vi "Restore Front Panel Window Position From File.vi"(8 "error in (no error)":errorcluster, 11 "Actor in":refnum<class "Actor.lvclass">) -> (0 "error out":errorcluster)   [LabVIEW 2021, in "Actor.lvclass"]
uses:
  Actor.lvclass
  Actor.lvclass/Actor.ctl
  <vilib>/Utility/miscctls.llb/LVRectTypeDef.ctl
  <userlib>/_OpenG.lib/variantconfig/variantconfig.llb/openg_variant_configuration_file.lvlib
  <vilib>/Utility/config.llb/NI_LVConfig.lvlib
  <userlib>/_OpenG.lib/file/file.llb/openg_file.lvlib
  <userlib>/_OpenG.lib/file/file.llb/File Exists - Scalar__ogtk.vi
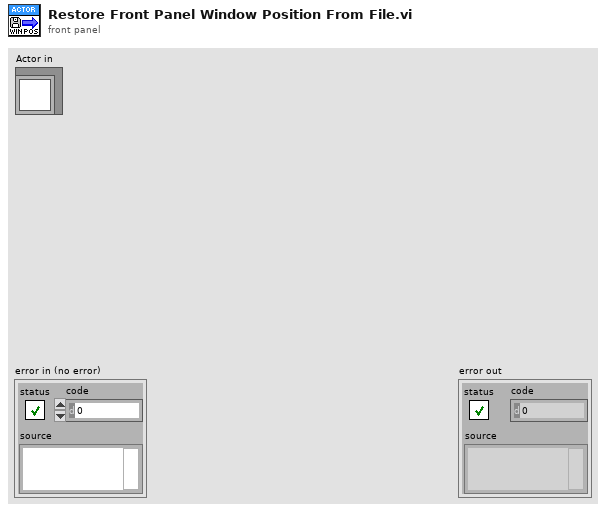
[diagram p1: front panel]
types:
  T1 = typedef "LVRectTypeDef.ctl" = cluster{"Left":i16, "Top":i16, "Right":i16, "Bottom":i16}
  T2 = typedef "NI_LVConfig.lvlib/Config Data RefNum.ctl" = refnum<k1>
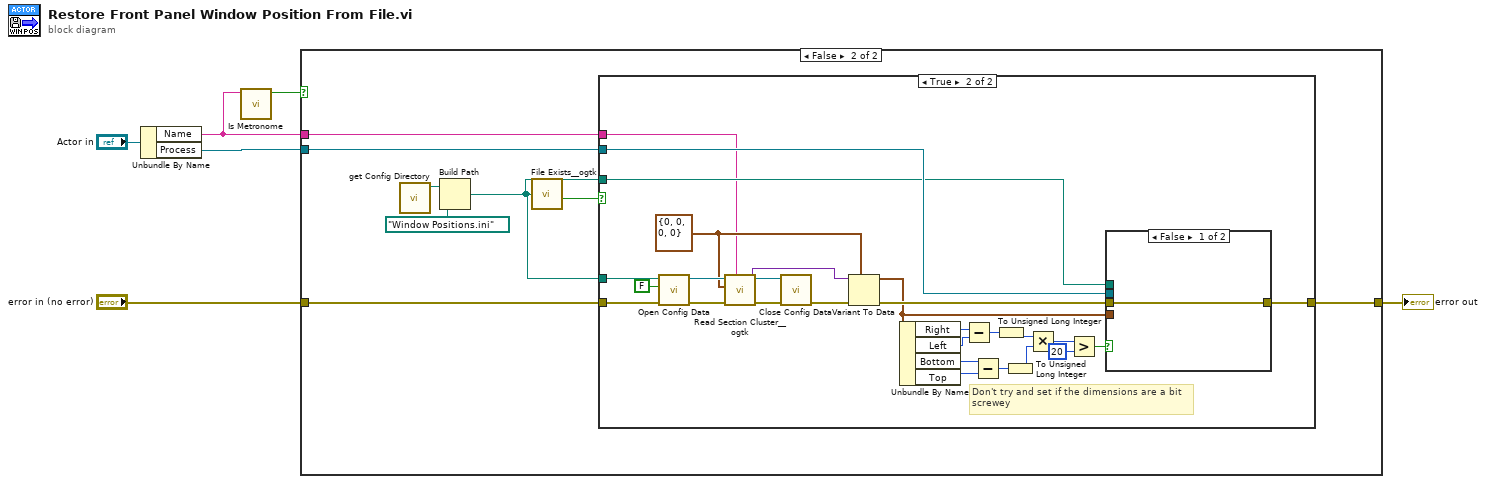
[diagram p0: block diagram]
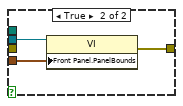
[diagram p4: hidden frame]
diagram:
  n1 = Unbundle By Name("Actor in") -> ("Name"=w1:string, "Process"=w5:refnum<vi>)
  n2 = call "Is Metronome.vi"("Actor Name"=w1) -> ("Is Metronome"=w2:bool)  [unwired: 10 in]
  n3 = case shown="False" w2 {
    tunnel: "error in (no error)" -> [w7 w9]
    tunnel: w5 -> [_ w15]
    tunnel: [w7 w13] -> w3
    tunnel: w1 -> [_ w8]
    frame True {
      # "Do not bother loading positions of Metronomes"
    }
    frame False {
      n4 = call "get Config Directory.vi"() -> ("Config Dir"=w10:path)  [unwired: 11 in]
      n5 = Build Path(base path=w10, name or relative path=path "Window Positions.ini" ("configuration file path")) -> (appended path=w11:path)
      n6 = call-poly <userlib>:"File Exists__ogtk.vi"("file path"=w11) -> ("exists"=w12:bool)  [unwired: 6 in, 1 out]
      n7 = case shown="True" w12 {
        tunnel: w9 -> [w16 w43]
        tunnel: w15 -> [_ w33]
        tunnel: [w16 w32] -> w13
        tunnel: w11 -> [_ w21]
        tunnel: w11 -> [_ w18]
        tunnel: w8 -> [_ w17]
        frame False {
        }
        frame True {
          w35 = T1 {"Left"=0, "Top"=0, "Right"=0, "Bottom"=0} ("Front Panel Window:Panel Bounds")
          # "Don't try and set if the dimensions are a bit screwey"
          n8 = call <vilib>:"Open Config Data.vi"("error in (no error)"=w43, "create file if necessary (T)"=FALSE, "configuration file path"=w21) -> ("error out"=w37:errorcluster, "refnum"=w38:T2)  [unwired: 6 in, 1 out]
          n9 = call <userlib>:"Read Section Cluster__ogtk.vi"("section (optional)"=w17, "error in (no error)"=w37, "Section Formatted Cluster Type"=w35, "refnum"=w38) -> ("error out"=w41:errorcluster, "Section Formatted Cluster"=w36:variant, "dup refnum"=w40:T2)  [unwired: 3 in, 2 out]
          n10 = call <vilib>:"Close Config Data.vi"("error in (no error)"=w41, "refnum"=w40) -> ("error out"=w42:errorcluster)  [unwired: 8 in, 1 out]
          n11 = Variant To Data(error in=w42, type=w35, Variant=w36) -> (data=w31:T1, error out=w34:errorcluster)
          n12 = Unbundle By Name(w31) -> ("Right"=w30:i16, "Left"=w29:i16, "Bottom"=w28:i16, "Top"=w27:i16)
          n13 = Subtract(x=w30, y=w29) -> (x-y=w26:i16)
          n14 = Subtract(x=w28, y=w27) -> (x-y=w25:i16)
          n15 = To Unsigned Long Integer(number=w26) -> (unsigned 32bit integer=w20:u32)
          n16 = To Unsigned Long Integer(number=w25) -> (unsigned 32bit integer=w19:u32)
          n17 = Multiply(x=w20, y=w19) -> (x*y=w24:u32)
          n18 = Greater?(x=w24, y=u32 20) -> (0:w22:bool)
          n19 = case shown="False" w22 {
            tunnel: w33 -> [_ w46]
            tunnel: [w44 w47] -> w32
            tunnel: w31 -> [_ w45]
            tunnel: w34 -> [w44 _]
            tunnel: w18 -> [_ _]
            frame False {
            }
            frame True {
              n20 = property class="VI"(reference=w46, "Front Panel.PanelBounds"=w45) -> (error out=w47:errorcluster)  [unwired: 1 in, 1 out]
            }
          }
        }
      }
    }
  }
  "error out" <- w3
